vi "Main.vi"() -> ()   [LabVIEW 2020]
uses:
  <vilib>/Instr/_visa.llb/VISA Find Search Mode.ctl
panel:
  in  "Exit":bool
  in  "Tab Control":T1(tab)
  out "Record Time [s]":ext format="%.2f"
  out "Meas. Periods Recorded":u32
  out "Target Directory":string
  out "Measurement Running":bool
  in  "Stop Recording":bool
  in  "Start Recording":bool
  in  "Measurement Name":string
  in  "Parent Directory":path
  in  "Export Channel 2":bool=TRUE
  in  "Export Channel 1":bool=TRUE
  in  "USB Device Address":string
  out "Meas. Periods to Process":u32
  out "Data Received [MB]":ext format="%.2f"
  in  "Disconnect":bool
  in  "Connect":bool
  out "Time Domain Plot":waveform(dbl)[](graph)=[{"t0"=timestamp(0 s since 1904-01-01), "dt"=3.90625e-06, "Y"=[]}, {"t0"=timestamp(0 s since 1904-01-01), "dt"=3.90625e-06, "Y"=[]}, {"t0"=timestamp(0 s since 1904-01-01), "dt"=3.90625e-06, "Y"=[]}, {"t0"=timestamp(0 s since 1904-01-01), "dt"=3.90625e-06, "Y"=[]}]
  in  "Remove DC Channel 1":bool=TRUE
  in  "Remove DC Channel 2":bool=TRUE
  in  "Measurement Period [ms]":u16=100 min=5 max=10000 step=5
  out "ENBW [Hz]":dbl
  in  "Weighting Mode":enum16{"Linear", "Exponential"}(ring)=enum."Exponential"
  out "Frequency Resolution [Hz]":dbl min=5.0 max=10000.0 step=5.0
  in  "Number of Averages":dbl=10.0
  out "Averaging Complete":bool
  in  "Restart Averaging":bool
  out "Averages Completed":dbl=1.0
  out "Frequency Domain Plot":cluster{"f0":dbl, "df":dbl, "magnitude":dbl[]}[](graph)=[{"f0"=0.0, "df"=inf, "magnitude"=[]}, {"f0"=0.0, "df"=inf, "magnitude"=[]}, {"f0"=0.0, "df"=inf, "magnitude"=[]}, {"f0"=0.0, "df"=inf, "magnitude"=[]}, {"f0"=0.0, "df"=10.0, "magnitude"=array[12800 elements]}, {"f0"=0.0, "df"=10.0, "magnitude"=array[12800 elements]}]
  in  "Averaging Mode":T2(ring)
  in  "Window":u16(ring)=1 items=["Rectangle"=0, "Hanning"=1, "Hamming"=2, "Blackman-Harris"=3, "Exact Blackman"=4, "Blackman"=5, "Flat Top"=6, "Triangle"=30, "Bartlett-Hanning"=31, "Welch"=34, "Kaiser"=60, "Gaussian"=62]
  in  "Spectrum Type":T3(ring)
  in  "Scaling Channel 2 [dB]":dbl
  in  "Scaling Channel 1 [dB]":dbl
  in  "Sample Rate [Hz]":u32=256000
  in  "Packet Size [Bytes]":u16=20480
  in  "Packet Length [ms]":u16=5
  in  "Voltage Conversion Factor [V]":dbl=6.55e-07
  # "NI VISA Data Connection"
  # "File Export"
  # "Status"
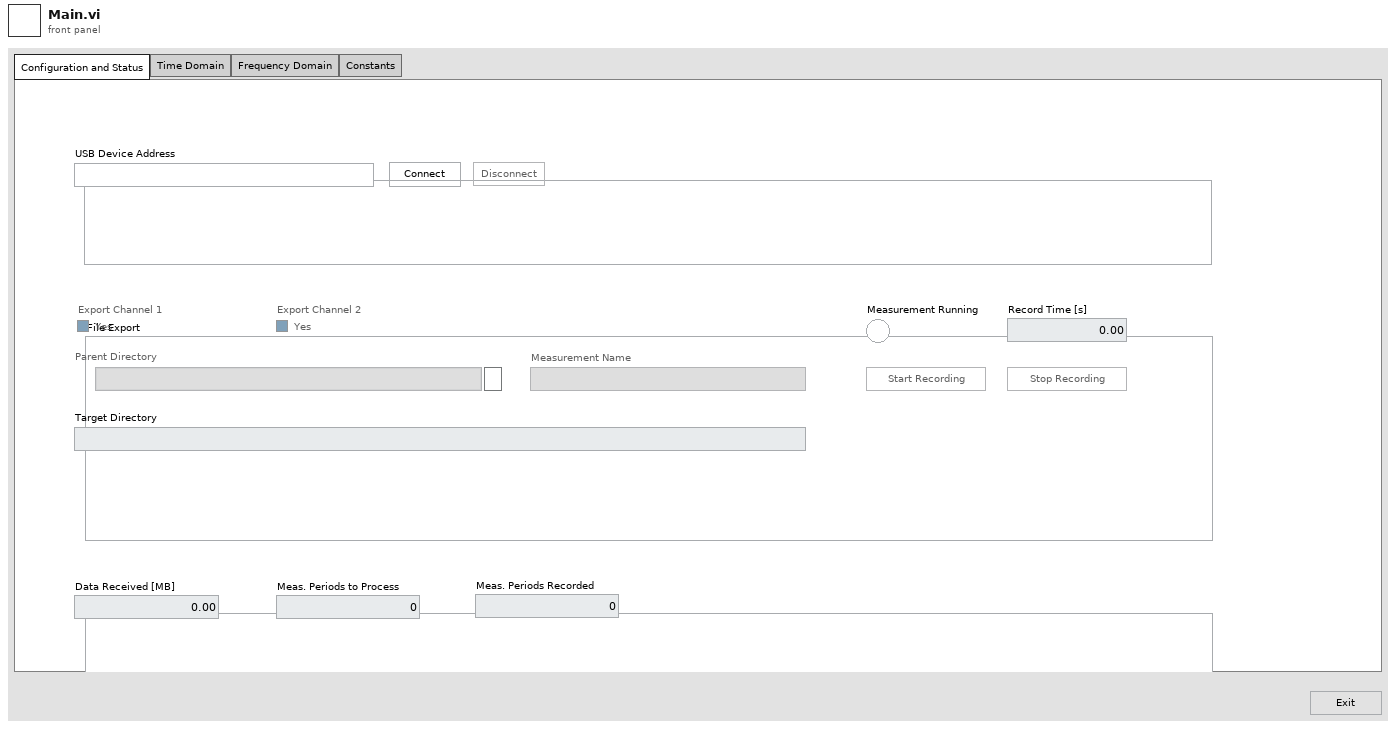
[diagram p1: front panel]
types:
  T1 = enum32{"Configuration and Status", "Time Domain", "Frequency Domain", "Constants"}
  T2 = enum16{"No averaging", "Vector averaging", "RMS averaging", "Peak hold"}
  T3 = enum16{"Amplitude Spectrum", "Amplitude Spectral Density"}
  T4 = enum8{"Enabled", "Disabled", "Disabled and Grayed Out"}
  T5 = typedef "VISA Find Search Mode.ctl" = u32
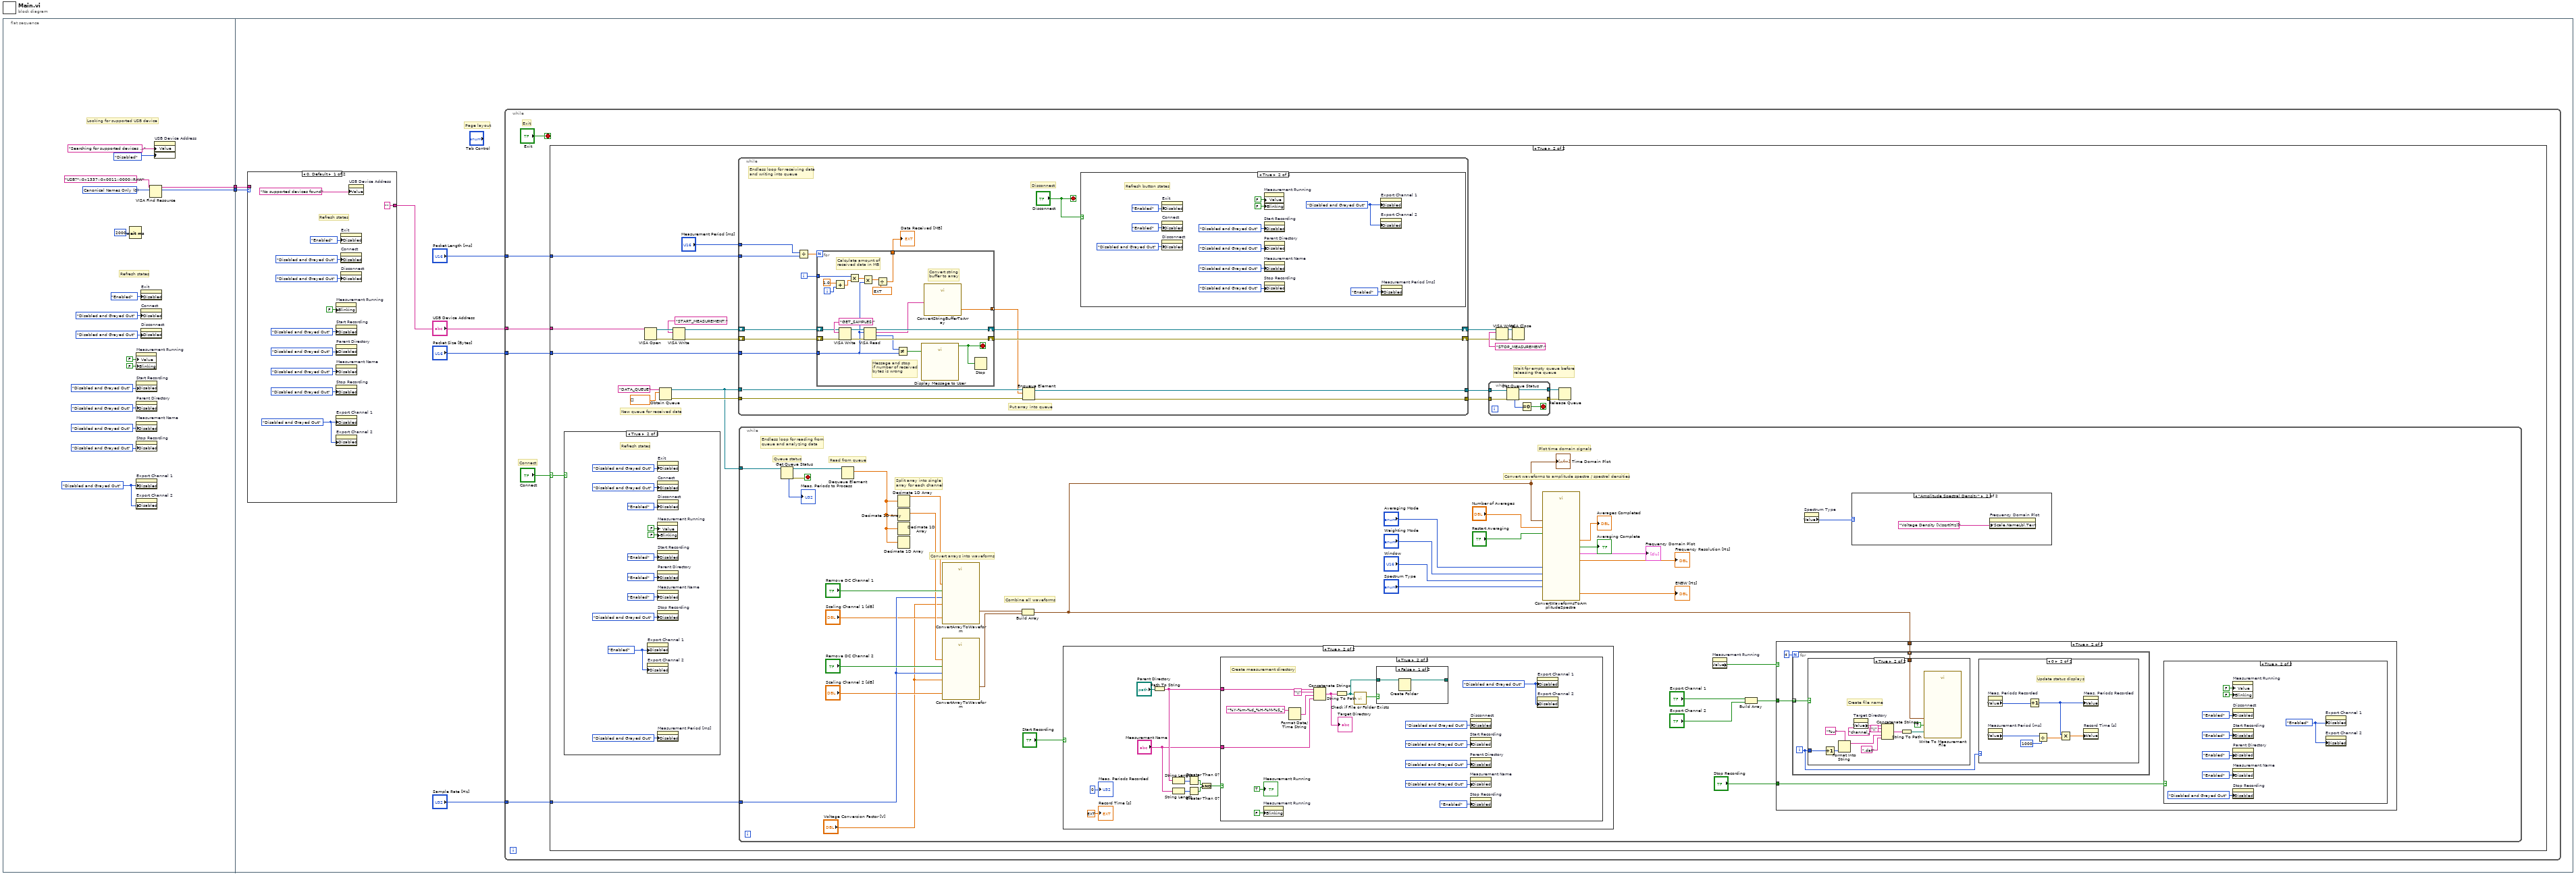
[diagram p0: block diagram]
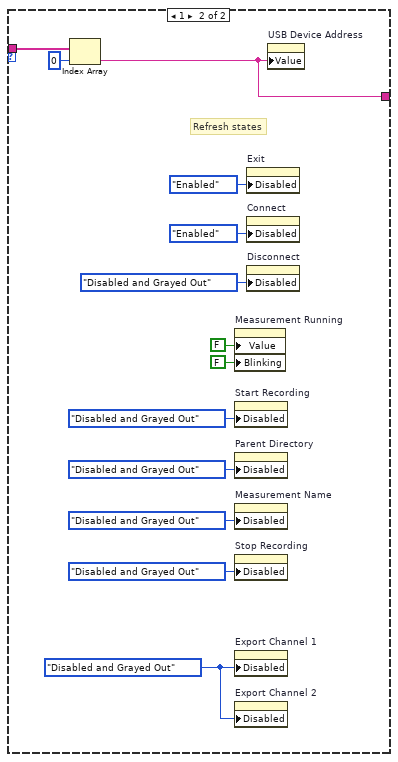
[diagram p2: hidden frame]
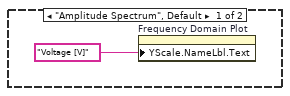
[diagram p4: hidden frame]
diagram:
  n1 = flat-sequence {
    tunnel: [w15] -> w2
    tunnel: [w14] -> w1
    tunnel: w2 -> [w22]
    tunnel: w1 -> [w21]
    frame #0 {
      w3 = T4."Disabled and Grayed Out" ("Disabled")
      w17 = T5 0 items=["Canonical Names Only"=0, "Aliases Only"=2, "Include Matching Aliases"=3, "Include All Aliases"=4] ("Search Mode")
      # "Refresh states"
      # "Looking for supported USB device"
      n2 = Wait (ms)(milliseconds to wait=u32 2000) -> ()  [unwired: 1 out]
      n3 = property on="Measurement Running" class="Bool (strict)"("Value"=FALSE ("Measurement Running"), "Blinking"=FALSE) -> ()  [unwired: 2 in, 2 out]
      n4 = property on="Start Recording" class="Bool"("Disabled"=T4."Disabled and Grayed Out") -> ()  [unwired: 2 in, 2 out]
      n5 = property on="Parent Directory" class="Path"("Disabled"=T4."Disabled and Grayed Out") -> ()  [unwired: 2 in, 2 out]
      n6 = property on="Measurement Name" class="Str"("Disabled"=T4."Disabled and Grayed Out") -> ()  [unwired: 2 in, 2 out]
      n7 = property on="Stop Recording" class="Bool"("Disabled"=T4."Disabled and Grayed Out") -> ()  [unwired: 2 in, 2 out]
      n8 = property on="Export Channel 1" class="Bool (strict)"("Disabled"=w3) -> ()  [unwired: 2 in, 2 out]
      n9 = property on="Export Channel 2" class="Bool (strict)"("Disabled"=w3) -> ()  [unwired: 2 in, 2 out]
      n10 = property on="Exit" class="Bool"("Disabled"=T4."Enabled") -> ()  [unwired: 2 in, 2 out]
      n11 = property on="Connect" class="Bool"("Disabled"=T4."Disabled and Grayed Out") -> ()  [unwired: 2 in, 2 out]
      n12 = property on="Disconnect" class="Bool"("Disabled"=T4."Disabled and Grayed Out") -> ()  [unwired: 2 in, 2 out]
      n13 = VISA Find Resource(10:w17, 11:"USB?*::0x1337::0x0011::0000::RAW" ("expression (\"?*\")")) -> (2:w15:u32, 3:w14:string[])  [unwired: 1 in, 1 out]
      n14 = property on="USB Device Address" class="Str"("Value"="Searching for supported devices ...", "DisabledEnum"=T4."Disabled" ("Disabled")) -> ()  [unwired: 2 in, 2 out]
    }
    frame #1 {
      # "Page layout"
      n15 = case shown="0, Default" w22 {
        tunnel: w21 -> [_ w49]
        tunnel: ["" w44] -> w20
        frame 0, Default {
          w26 = T4."Disabled and Grayed Out" ("Disabled")
          # "Refresh states"
          n16 = property on="Measurement Running" class="Bool (strict)"("Blinking"=FALSE) -> ()  [unwired: 2 in, 2 out]
          n17 = property on="Start Recording" class="Bool"("Disabled"=T4."Disabled and Grayed Out") -> ()  [unwired: 2 in, 2 out]
          n18 = property on="Parent Directory" class="Path"("Disabled"=T4."Disabled and Grayed Out") -> ()  [unwired: 2 in, 2 out]
          n19 = property on="Measurement Name" class="Str"("Disabled"=T4."Disabled and Grayed Out") -> ()  [unwired: 2 in, 2 out]
          n20 = property on="Stop Recording" class="Bool"("Disabled"=T4."Disabled and Grayed Out") -> ()  [unwired: 2 in, 2 out]
          n21 = property on="Export Channel 1" class="Bool (strict)"("Disabled"=w26) -> ()  [unwired: 2 in, 2 out]
          n22 = property on="Export Channel 2" class="Bool (strict)"("Disabled"=w26) -> ()  [unwired: 2 in, 2 out]
          n23 = property on="Exit" class="Bool"("Disabled"=T4."Enabled") -> ()  [unwired: 2 in, 2 out]
          n24 = property on="Connect" class="Bool"("Disabled"=T4."Disabled and Grayed Out") -> ()  [unwired: 2 in, 2 out]
          n25 = property on="Disconnect" class="Bool"("Disabled"=T4."Disabled and Grayed Out") -> ()  [unwired: 2 in, 2 out]
          n26 = property on="USB Device Address" class="Str"("Value"="No supported devices found") -> ()  [unwired: 2 in, 2 out]
        }
        frame 1 {
          w37 = T4."Disabled and Grayed Out" ("Disabled")
          # "Refresh states"
          n27 = Index Array(array=w49, index=0) -> (element=w44:string)
          n28 = property on="Measurement Running" class="Bool (strict)"("Value"=FALSE ("Measurement Running"), "Blinking"=FALSE) -> ()  [unwired: 2 in, 2 out]
          n29 = property on="Start Recording" class="Bool"("Disabled"=T4."Disabled and Grayed Out") -> ()  [unwired: 2 in, 2 out]
          n30 = property on="Parent Directory" class="Path"("Disabled"=T4."Disabled and Grayed Out") -> ()  [unwired: 2 in, 2 out]
          n31 = property on="Measurement Name" class="Str"("Disabled"=T4."Disabled and Grayed Out") -> ()  [unwired: 2 in, 2 out]
          n32 = property on="Stop Recording" class="Bool"("Disabled"=T4."Disabled and Grayed Out") -> ()  [unwired: 2 in, 2 out]
          n33 = property on="Export Channel 1" class="Bool (strict)"("Disabled"=w37) -> ()  [unwired: 2 in, 2 out]
          n34 = property on="Export Channel 2" class="Bool (strict)"("Disabled"=w37) -> ()  [unwired: 2 in, 2 out]
          n35 = property on="Exit" class="Bool"("Disabled"=T4."Enabled") -> ()  [unwired: 2 in, 2 out]
          n36 = property on="Connect" class="Bool"("Disabled"=T4."Enabled") -> ()  [unwired: 2 in, 2 out]
          n37 = property on="Disconnect" class="Bool"("Disabled"=T4."Disabled and Grayed Out") -> ()  [unwired: 2 in, 2 out]
          n38 = property on="USB Device Address" class="Str"("Value"=w44) -> ()  [unwired: 2 in, 2 out]
        }
      }
      n39 = while {
        tunnel: "Packet Size [Bytes]" -> [w54]
        tunnel: w20 -> [w53]
        tunnel: "Packet Length [ms]" -> [w52]
        tunnel: "Sample Rate [Hz]" -> [w51]
        stop <- "Exit" stop-if-true
        # "Exit"
        # "Connect"
        n40 = case shown="True" "Connect" {
          selector: "Connect" -> [_ w66]
          tunnel: w53 -> [_ w69]
          tunnel: w54 -> [_ w68]
          tunnel: w52 -> [_ w67]
          tunnel: w51 -> [_ w61]
          frame False {
          }
          frame True {
            # "Wait for empty queue before\nreleasing the queue"
            # "New queue for received data"
            n41 = case shown="True" w66 {
              frame False {
              }
              frame True {
                w185 = T4."Enabled" ("Disabled")
                # "Refresh states"
                n42 = property on="Export Channel 1" class="Bool (strict)"("Disabled"=w185) -> ()  [unwired: 2 in, 2 out]
                n43 = property on="Export Channel 2" class="Bool (strict)"("Disabled"=w185) -> ()  [unwired: 2 in, 2 out]
                n44 = property on="Exit" class="Bool"("Disabled"=T4."Disabled and Grayed Out") -> ()  [unwired: 2 in, 2 out]
                n45 = property on="Connect" class="Bool"("Disabled"=T4."Disabled and Grayed Out") -> ()  [unwired: 2 in, 2 out]
                n46 = property on="Disconnect" class="Bool"("Disabled"=T4."Enabled") -> ()  [unwired: 2 in, 2 out]
                n47 = property on="Measurement Running" class="Bool (strict)"("Value"=FALSE ("Measurement Running"), "Blinking"=FALSE) -> ()  [unwired: 2 in, 2 out]
                n48 = property on="Start Recording" class="Bool"("Disabled"=T4."Enabled") -> ()  [unwired: 2 in, 2 out]
                n49 = property on="Parent Directory" class="Path"("Disabled"=T4."Enabled") -> ()  [unwired: 2 in, 2 out]
                n50 = property on="Measurement Name" class="Str"("Disabled"=T4."Enabled") -> ()  [unwired: 2 in, 2 out]
                n51 = property on="Stop Recording" class="Bool"("Disabled"=T4."Disabled and Grayed Out") -> ()  [unwired: 2 in, 2 out]
                n52 = property on="Measurement Period [ms]" class="DigNum (strict)"("Disabled"=T4."Disabled and Grayed Out") -> ()  [unwired: 2 in, 2 out]
              }
            }
            n53 = VISA Open(VISA resource name=w69) -> (VISA resource name=w78:refnum<visa-resource-name>, error out=w79:errorcluster)  [unwired: 1 in, 3 out]
            n54 = Obtain Queue(name (unnamed)="DATA_QUEUE", element data type=dbl[] [] ("Output Array")) -> (queue out=w62:refnum<queue>, error out=w63:errorcluster)  [unwired: 3 in, 1 out]
            n55 = VISA Write(VISA resource name=w78, write buffer="START_MEASUREMENT;", error in (no error)=w79) -> (VISA resource name out=w76:refnum<visa-resource-name>, error out=w75:errorcluster)  [unwired: 1 out]
            n56 = while {
              shift-right: [w208] -> w74
              shift-left: w76 -> [w210]
              shift-right: [w207] -> w70
              shift-left: w75 -> [w209]
              tunnel: w68 -> [w204]
              tunnel: w67 -> [w205]
              tunnel: w63 -> [w199]
              tunnel: w62 -> [w202]
              tunnel: [w197] -> w60
              tunnel: [w196] -> w59
              tunnel: "Measurement Period [ms]" -> [w195]
              i -> [w198]
              stop <- "Disconnect" stop-if-true
              # "Endless loop for receiving data\nand writing into queue"
              # "Put array into queue"
              # "Disconnect"
              n57 = Divide(x=w195, y=w205) -> (x/y=w206:dbl)
              n58 = for {
                N: w206 -> [_]
                shift-right: [w237] -> w208
                shift-left: w210 -> [w241]
                shift-right: [w236] -> w207
                shift-left: w209 -> [w240]
                tunnel: w198 -> [w234]
                tunnel: w204 -> [w224]
                tunnel: [w230] -> w203
                tunnel: [w226] -> w201 mode=concatenating
                i -> [w227]
                stop <- w222 stop-if-true
                # "Message and stop\nif number of received\nbytes is wrong"
                # "Convert string\nbuffer to array"
                # "Calculate amount of\nreceived data in MB"
                n59 = Add(x=1.0, y=w227) -> (x+y=w229:dbl)
                n60 = VISA Write(VISA resource name=w241, write buffer="GET_SAMPLES;" ("write buffer 2"), error in (no error)=w240) -> (VISA resource name out=w238:refnum<visa-resource-name>, error out=w239:errorcluster)  [unwired: 1 out]
                n61 = Multiply(x=w234, y=w229) -> (x*y=w233:ext)
                n62 = Multiply(x=w233, y=w224) -> (x*y=w232:ext)
                n63 = VISA Read(VISA resource name=w238, byte count=w224, error in (no error)=w239) -> (VISA resource name out=w237:refnum<visa-resource-name>, read buffer=w235:string, return count=w225:u32, error out=w236:errorcluster)
                n64 = Divide(x=w232, y=ext 1000000.0) -> (x/y=w230:ext)
                n65 = Not Equal?(x=w225, y=w224) -> (x != y?=w223:bool)
                n66 = call "Display Message to User"("Enable"=w223) -> ("Exit"=w222:bool)  [unwired: 9 in, 1 out]
                n67 = call "ConvertStringBufferToArray.vi"("Input String Buffer"=w235) -> ("Output Array"=w226:dbl[])  [unwired: 10 in]
                n68 = Stop(stop? (T)=w222) -> ()
              }
              "Data Received [MB]" <- w203
              n69 = Enqueue Element(queue=w202, element=w201, error in (no error)=w199) -> (queue out=w197:refnum<queue>, error out=w196:errorcluster)  [unwired: 1 in, 1 out]
              n70 = case shown="True" "Disconnect" {
                frame False {
                }
                frame True {
                  w212 = T4."Disabled and Grayed Out" ("Disabled")
                  # "Refresh button states"
                  n71 = property on="Exit" class="Bool"("Disabled"=T4."Enabled") -> ()  [unwired: 2 in, 2 out]
                  n72 = property on="Connect" class="Bool"("Disabled"=T4."Enabled") -> ()  [unwired: 2 in, 2 out]
                  n73 = property on="Disconnect" class="Bool"("Disabled"=T4."Disabled and Grayed Out") -> ()  [unwired: 2 in, 2 out]
                  n74 = property on="Measurement Running" class="Bool (strict)"("Value"=FALSE ("Measurement Running"), "Blinking"=FALSE) -> ()  [unwired: 2 in, 2 out]
                  n75 = property on="Start Recording" class="Bool"("Disabled"=T4."Disabled and Grayed Out") -> ()  [unwired: 2 in, 2 out]
                  n76 = property on="Parent Directory" class="Path"("Disabled"=T4."Disabled and Grayed Out") -> ()  [unwired: 2 in, 2 out]
                  n77 = property on="Measurement Name" class="Str"("Disabled"=T4."Disabled and Grayed Out") -> ()  [unwired: 2 in, 2 out]
                  n78 = property on="Stop Recording" class="Bool"("Disabled"=T4."Disabled and Grayed Out") -> ()  [unwired: 2 in, 2 out]
                  n79 = property on="Export Channel 1" class="Bool (strict)"("Disabled"=w212) -> ()  [unwired: 2 in, 2 out]
                  n80 = property on="Export Channel 2" class="Bool (strict)"("Disabled"=w212) -> ()  [unwired: 2 in, 2 out]
                  n81 = property on="Measurement Period [ms]" class="DigNum (strict)"("Disabled"=T4."Enabled") -> ()  [unwired: 2 in, 2 out]
                }
              }
            }
            n82 = while {
              tunnel: w62 -> [w118]
              tunnel: w61 -> [w113]
              stop <- w108 stop-if-true
              # "Combine all waveforms"
              # "Convert waveforms to amplitude spectra / spectral densities"
              # "Endless loop for reading from\nqueue and analyzing data"
              # "Plot time domain signals"
              # "Convert arrays into waveforms"
              # "Split array into single\narray for each channel"
              # "Read from queue"
              # "Queue status"
              n83 = Get Queue Status(queue=w118) -> (queue out=w109:refnum<queue>, error out=w108:errorcluster, # elements in queue=→"Meas. Periods to Process":i32)  [unwired: 2 in, 5 out]
              n84 = Dequeue Element(queue=w109) -> (element=w98:dbl[])  [unwired: 2 in, 3 out]
              n85 = Decimate 1D Array(w98) -> (w115:dbl[])  [unwired: 3 out]
              n86 = Decimate 1D Array(w98) -> (w114:dbl[])  [unwired: 3 out]
              n87 = Decimate 1D Array(w98) -> ()  [unwired: 4 out]
              n88 = Decimate 1D Array(w98) -> ()  [unwired: 4 out]
              n89 = call "ConvertArrayToWaveform.vi"("Scaling [dB]"="Scaling Channel 1 [dB]", "Remove DC"="Remove DC Channel 1", "Input Array"=w115, "Voltage Conversion Factor [V]"="Voltage Conversion Factor [V]", "Sample Rate [Hz]"=w113) -> ("Output Waveform"=w107:waveform(dbl))  [unwired: 6 in]
              n90 = call "ConvertArrayToWaveform.vi"("Scaling [dB]"="Scaling Channel 2 [dB]", "Remove DC"="Remove DC Channel 2", "Input Array"=w114, "Voltage Conversion Factor [V]"="Voltage Conversion Factor [V]", "Sample Rate [Hz]"=w113) -> ("Output Waveform"=w106:waveform(dbl))  [unwired: 6 in]
              n91 = Build Array(w107, w106) -> (w96:waveform(dbl)[])
              "Time Domain Plot" <- w96
              n92 = case shown="True" "Start Recording" {
                frame False {
                }
                frame True {
                  n93 = Path To String(path="Parent Directory") -> (string=w163:string)
                  n94 = String Length(string=w163) -> (length=w161:i32)
                  n95 = String Length(string="Measurement Name") -> (length=w160:i32)
                  n96 = Greater Than 0?(x=w161) -> (x > 0?=w159:bool)
                  n97 = Greater Than 0?(x=w160) -> (x > 0?=w158:bool)
                  n98 = And(x=w159, y=w158) -> (x .and. y?=w157:bool)
                  n99 = case shown="True" w157 {
                    tunnel: w163 -> [_ w180]
                    tunnel: "Measurement Name" -> [_ w174]
                    frame False {
                    }
                    frame True {
                      w165 = T4."Disabled and Grayed Out" ("Disabled")
                      # "Create measurement directory"
                      n100 = property on="Measurement Running" class="Bool (strict)"("Blinking"=FALSE) -> ()  [unwired: 2 in, 2 out]
                      n101 = Format Date/Time String(time format string (%c)="%Y-%m-%d_%H-%M-%S_") -> (date/time string=w175:string)  [unwired: 2 in]
                      n102 = Concatenate Strings(w180, "\\" ("string"), w175, w174) -> (w167:string)
                      "Target Directory" <- w167
                      n103 = String To Path(string=w167) -> (path=w177:path)
                      n104 = call <vilib>:"Check if File or Folder Exists.vi"("path"=w177) -> ("file or folder exists?"=w178:bool)  [unwired: 8 in, 2 out]
                      n105 = case shown="False" w178 {
                        tunnel: w177 -> [w182 w183]
                        tunnel: [w181 w183] -> _
                        frame False {
                          n106 = Create Folder(path (use dialog)=w182) -> (created path=w181:path)  [unwired: 2 in, 2 out]
                        }
                        frame True {
                        }
                      }
                      n107 = property on="Start Recording" class="Bool"("Disabled"=T4."Disabled and Grayed Out") -> ()  [unwired: 2 in, 2 out]
                      n108 = property on="Parent Directory" class="Path"("Disabled"=T4."Disabled and Grayed Out") -> ()  [unwired: 2 in, 2 out]
                      n109 = property on="Measurement Name" class="Str"("Disabled"=T4."Disabled and Grayed Out") -> ()  [unwired: 2 in, 2 out]
                      n110 = property on="Stop Recording" class="Bool"("Disabled"=T4."Enabled") -> ()  [unwired: 2 in, 2 out]
                      n111 = property on="Disconnect" class="Bool"("Disabled"=T4."Disabled and Grayed Out") -> ()  [unwired: 2 in, 2 out]
                      n112 = property on="Export Channel 1" class="Bool (strict)"("Disabled"=w165) -> ()  [unwired: 2 in, 2 out]
                      n113 = property on="Export Channel 2" class="Bool (strict)"("Disabled"=w165) -> ()  [unwired: 2 in, 2 out]
                      "Measurement Running" <- TRUE
                    }
                  }
                  "Meas. Periods Recorded" <- u32 0 ("Meas. Periods Recorded")
                  "Record Time [s]" <- ext 0.0 ("Record Time [s]")
                }
              }
              n114 = call "ConvertWaveformsToAmplitudeSpectra.vi"("Averaging Mode"="Averaging Mode", "Number of Averages"="Number of Averages", "Weighting Mode"="Weighting Mode", "Export Mode"="Spectrum Type", "Waveforms"=w96, "Window"="Window", "Restart Averaging"="Restart Averaging") -> ("Frequency Resolution [Hz]"=→"Frequency Resolution [Hz]":dbl, "Amplitude Spectral Density"=→"Frequency Domain Plot":cluster{"f0":dbl, "df":dbl, "magnitude":dbl[]}[], "Averages Completed"=→"Averages Completed":dbl, "Averaging Done"=→"Averaging Complete":bool, "ENBW [Hz]"=→"ENBW [Hz]":dbl)
              n115 = property on="Measurement Running" class="Bool (strict)"() -> ("Value"=w102:bool)  [unwired: 2 in, 2 out]
              n116 = Build Array("Export Channel 1", "Export Channel 2") -> (w100:bool[])
              n117 = case shown="True" w102 {
                tunnel: "Stop Recording" -> [_ w125]
                tunnel: w100 -> [_ w124]
                tunnel: w96 -> [_ w122]
                frame False {
                }
                frame True {
                  n118 = for {
                    N: 4 -> [_]
                    tunnel: w124 -> [w128] mode=indexing
                    tunnel: w122 -> [w127] mode=indexing
                    i -> [w126]
                    n119 = case shown="True" w128 {
                      tunnel: w126 -> [_ w142]
                      tunnel: w127 -> [_ w136]
                      frame False {
                      }
                      frame True {
                        # "Create file name"
                        n120 = Increment(x=w142) -> (x+1=w141:i32)
                        n121 = Format Into String(format string="%u", w141) -> (resulting string=w139:string)  [unwired: 2 in, 1 out]
                        n122 = property on="Target Directory" class="Str"() -> ("Value"=w144:string)  [unwired: 2 in, 2 out]
                        n123 = Concatenate Strings(w144, "\\" ("string"), "channel_" ("string"), w139, ".dat" ("string")) -> (w143:string)
                        n124 = String To Path(string=w143) -> (path=w137:path)
                        n125 = call "Write To Measurement File"("Signals"=w136, "Enable"=TRUE, "Filename"=w137) -> ()  [unwired: 14 in, 3 out]
                      }
                    }
                    n126 = case shown="0" w126 {
                      frame -1, Default {
                      }
                      frame 0 {
                        # "Update status displays"
                        n127 = property on="Meas. Periods Recorded" class="DigNum (strict)"() -> ("Value"=w131:u32)  [unwired: 2 in, 2 out]
                        n128 = property on="Measurement Period [ms]" class="DigNum (strict)"() -> ("Value"=w133:u16)  [unwired: 2 in, 2 out]
                        n129 = Increment(x=w131) -> (x+1=w130:u32)
                        n130 = Divide(x=w133, y=u16 1000) -> (x/y=w134:dbl)
                        n131 = Multiply(x=w130, y=w134) -> (x*y=w129:dbl)
                        n132 = property on="Meas. Periods Recorded" class="DigNum (strict)"("Value"=w130) -> ()  [unwired: 2 in, 2 out]
                        n133 = property on="Record Time [s]" class="DigNum (strict)"("Value"=w129) -> ()  [unwired: 2 in, 2 out]
                      }
                    }
                  }
                  n134 = case shown="True" w125 {
                    frame False {
                    }
                    frame True {
                      w147 = T4."Enabled" ("Disabled")
                      n135 = property on="Measurement Running" class="Bool (strict)"("Value"=FALSE ("Measurement Running"), "Blinking"=FALSE) -> ()  [unwired: 2 in, 2 out]
                      n136 = property on="Disconnect" class="Bool"("Disabled"=T4."Enabled") -> ()  [unwired: 2 in, 2 out]
                      n137 = property on="Start Recording" class="Bool"("Disabled"=T4."Enabled") -> ()  [unwired: 2 in, 2 out]
                      n138 = property on="Parent Directory" class="Path"("Disabled"=T4."Enabled") -> ()  [unwired: 2 in, 2 out]
                      n139 = property on="Measurement Name" class="Str"("Disabled"=T4."Enabled") -> ()  [unwired: 2 in, 2 out]
                      n140 = property on="Stop Recording" class="Bool"("Disabled"=T4."Disabled and Grayed Out") -> ()  [unwired: 2 in, 2 out]
                      n141 = property on="Export Channel 1" class="Bool (strict)"("Disabled"=w147) -> ()  [unwired: 2 in, 2 out]
                      n142 = property on="Export Channel 2" class="Bool (strict)"("Disabled"=w147) -> ()  [unwired: 2 in, 2 out]
                    }
                  }
                }
              }
              n143 = property on="Spectrum Type" class="Enum (strict)"() -> ("Value"=w89:T3)  [unwired: 2 in, 2 out]
              n144 = case shown="\"Amplitude Spectral Density\"" w89 {
                frame "Amplitude Spectrum", Default {
                  n145 = property on="Frequency Domain Plot" class="WFGraph (strict)"("YScale.NameLbl.Text"="Voltage [V]" ("Y Scale.Name Label.Text")) -> ()  [unwired: 2 in, 2 out]
                }
                frame "Amplitude Spectral Density" {
                  n146 = property on="Frequency Domain Plot" class="WFGraph (strict)"("YScale.NameLbl.Text"="Voltage Density [V/sqrt(Hz)]" ("Y Scale.Name Label.Text")) -> ()  [unwired: 2 in, 2 out]
                }
              }
            }
            n147 = while {
              tunnel: w60 -> [w85]
              tunnel: w59 -> [w84]
              tunnel: [w81] -> w58
              tunnel: [w80] -> w57
              stop <- w83 stop-if-true
              n148 = Get Queue Status(queue=w85, error in (no error)=w84) -> (queue out=w81:refnum<queue>, error out=w80:errorcluster, # elements in queue=w82:i32)  [unwired: 1 in, 5 out]
              n149 = Equal To 0?(x=w82) -> (x = 0?=w83:bool)
            }
            n150 = VISA Write(VISA resource name=w74, write buffer="STOP_MEASUREMENT;" ("write buffer 3"), error in (no error)=w70) -> (VISA resource name out=w72:refnum<visa-resource-name>, error out=w73:errorcluster)  [unwired: 1 out]
            n151 = VISA Close(VISA resource name=w72, error in (no error)=w73) -> ()  [unwired: 1 out]
            n152 = Release Queue(queue=w58, error in (no error)=w57) -> ()  [unwired: 1 in, 3 out]
          }
        }
      }
    }
  }
